vi "ACTION.vi"(8 "error in (no error)":errorcluster, 9 "STEP State":T1, 10 "CORE":refnum<queue>, 11 "Scale Calibration in":refnum<class "Scale Calibration.lvclass">) -> (0 "error out":errorcluster, 3 "Scale Calibration out":refnum<class "Scale Calibration.lvclass">)   [LabVIEW 2014, in "SeqLoop.lvlib" / "STEP Classes.lvlib" / "Scale Calibration.lvclass"]
uses:
  Scale Calibration.lvclass
  TypeDefs/STEP State.ctl
  APIs/Message Queue/Message Cluster.ctl
  Scale Calibration.lvclass/Scale Calibration.ctl
  APIs/Message Queue/Enqueue Message (Array).vi
  APIs/Message Queue/Enqueue Message (Single).vi
  APIs/Message Queue/WINFAS 2 Message Queue.lvlib
  SeqLoop.lvlib
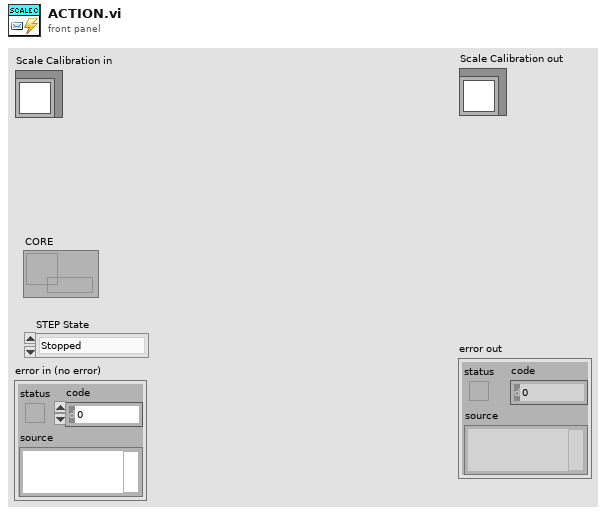
[diagram p1: front panel]
types:
  T1 = typedef "SeqLoop.lvlib/STEP State.ctl" = enum16{"Stopped", "First Call", "Idle...", "Advance OK", "Alarm", "Output Security", "Error"}
  T2 = cluster{"HWSync 1":bool, "HWSync 2":bool, "HWSync 3":bool, "HWSync 4":bool, "HWSync 5":bool}
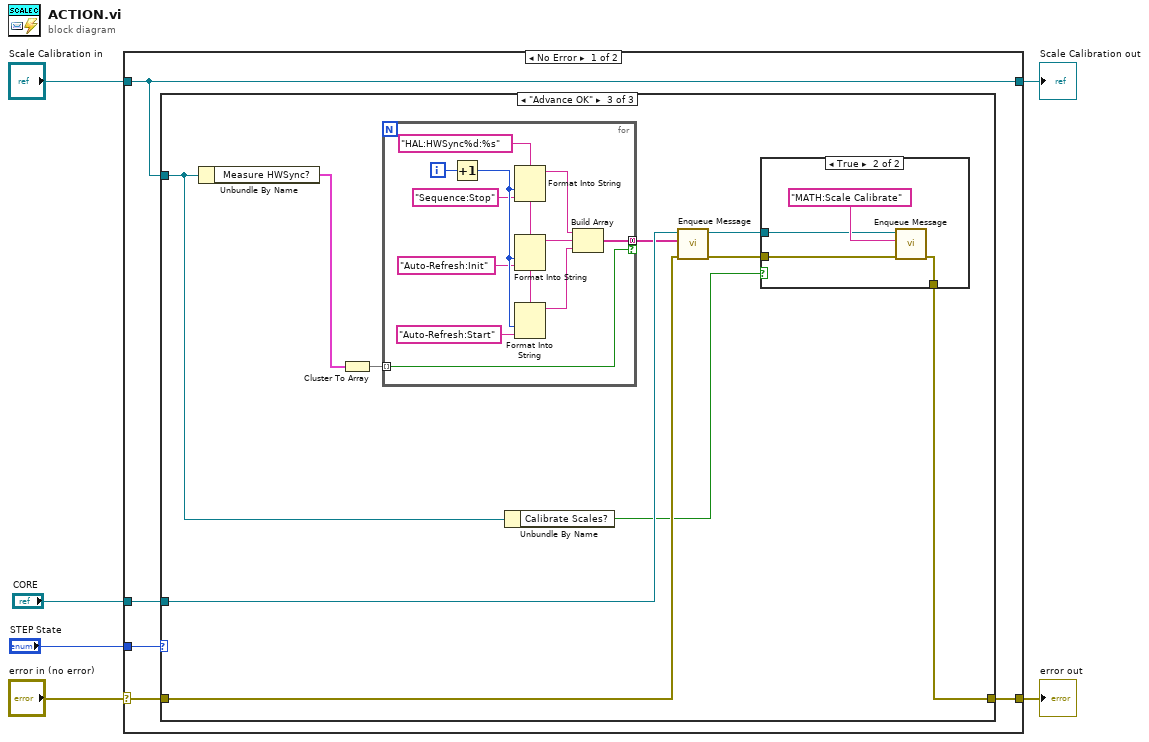
[diagram p0: block diagram]
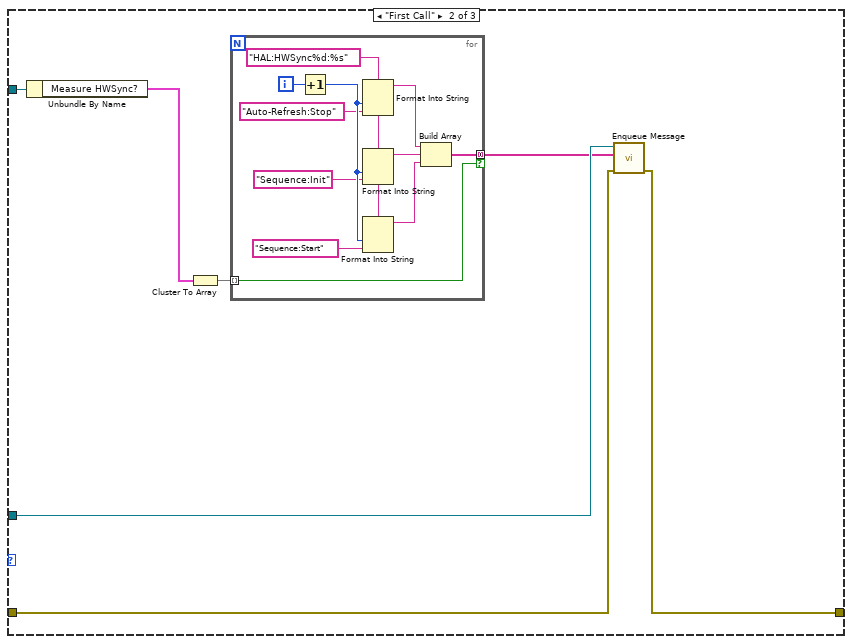
[diagram p3: hidden frame]
diagram:
  n1 = case shown="No Error" "error in (no error)" {
    selector: "error in (no error)" -> [w8 w58]
    tunnel: [w7 w58] -> w3
    tunnel: [w9 w57] -> w5
    tunnel: "Scale Calibration in" -> [w9 w57]
    tunnel: "CORE" -> [w10 _]
    tunnel: "STEP State" -> [w11 _]
    frame No Error {
      n2 = case shown="\"Advance OK\"" w11 {
        tunnel: w10 -> [_ w16 w38]
        tunnel: w9 -> [_ w18 w32]
        tunnel: w8 -> [w12 w15 w37]
        tunnel: [w12 w14 w34] -> w7
        frame Default {
        }
        frame "First Call" {
          n3 = Unbundle By Name(w18) -> ("Measure HWSync?"=w17:T2)
          n4 = Cluster To Array(cluster=w17) -> (array=w19:bool[])
          n5 = for {
            tunnel: w19 -> [w20] mode=indexing
            tunnel: [w21] -> w13 mode=concatenating if=w20
            i -> [w30]
            w29 = "HAL:HWSync%d:%s" ("format string")
            n6 = Increment(x=w30) -> (x+1=w28:i32)
            n7 = Format Into String(format string=w29, w28, "Auto-Refresh:Stop" ("format string")) -> (resulting string=w24:string)  [unwired: 2 in, 1 out]
            n8 = Format Into String(format string=w29, w28, "Sequence:Init" ("format string")) -> (resulting string=w23:string)  [unwired: 2 in, 1 out]
            n9 = Format Into String(format string=w29, w28, "Sequence:Start" ("format string")) -> (resulting string=w22:string)  [unwired: 2 in, 1 out]
            n10 = Build Array(w24, w23, w22) -> (w21:string[])
          }
          n11 = call-poly "Enqueue Message.vi"("error in (no error)"=w15, "Message Array"=w13, "Message Queue"=w16) -> ("error out"=w14:errorcluster)  [unwired: 7 in, 1 out]
        }
        frame "Advance OK" {
          n12 = Unbundle By Name(w32) -> ("Measure HWSync?"=w39:T2)
          n13 = Cluster To Array(cluster=w39) -> (array=w40:bool[])
          n14 = for {
            tunnel: w40 -> [w46] mode=indexing
            tunnel: [w47] -> w36 mode=concatenating if=w46
            i -> [w56]
            w55 = "HAL:HWSync%d:%s" ("format string")
            n15 = Increment(x=w56) -> (x+1=w54:i32)
            n16 = Format Into String(format string=w55, w54, "Sequence:Stop" ("format string")) -> (resulting string=w50:string)  [unwired: 2 in, 1 out]
            n17 = Format Into String(format string=w55, w54, "Auto-Refresh:Init" ("format string")) -> (resulting string=w49:string)  [unwired: 2 in, 1 out]
            n18 = Format Into String(format string=w55, w54, "Auto-Refresh:Start" ("format string")) -> (resulting string=w48:string)  [unwired: 2 in, 1 out]
            n19 = Build Array(w50, w49, w48) -> (w47:string[])
          }
          n20 = Unbundle By Name(w32) -> ("Calibrate Scales?"=w31:bool)
          n21 = call-poly "Enqueue Message.vi"("error in (no error)"=w37, "Message Array"=w36, "Message Queue"=w38) -> ("error out"=w35:errorcluster, "dup Message Queue"=w33:refnum<queue>)  [unwired: 7 in]
          n22 = case shown="True" w31 {
            tunnel: w35 -> [w41 w45]
            tunnel: [w41 w44] -> w34
            tunnel: w33 -> [_ w42]
            frame False {
            }
            frame True {
              n23 = call-poly "Enqueue Message.vi"("error in (no error)"=w45, "Message"="MATH:Scale Calibrate" ("format string"), "Message Queue"=w42) -> ("error out"=w44:errorcluster)  [unwired: 7 in, 1 out]
            }
          }
        }
      }
    }
    frame Error {
    }
  }
  "error out" <- w3
  "Scale Calibration out" <- w5
